vi "tcsWEP_logEvent_loopTimeOutOfRange.vi"(8 "error in (no error)":errorcluster, 11 "logevent_loopTimeOutOfRange_Ctl":T1) -> (0 "error out":errorcluster, 2 "function return":i32, 3 "logevent_loopTimeOutOfRange_Ctl out":T1)   [LabVIEW 2016, in "SALLV_tcsWEP.lvlib"]
doc: "int tcsWEP_shm_logEvent_loopTimeOutOfRangeLV(tcsWEP_logevent_loopTimeOutOfRangeLV *logevent_loopTimeOutOfRange_Ctl );"
uses:
  SALLV_tcsWEP.lvlib
  DataTypes/logevent_loopTimeOutOfRange.ctl
  SALLV_tcsWEP.so
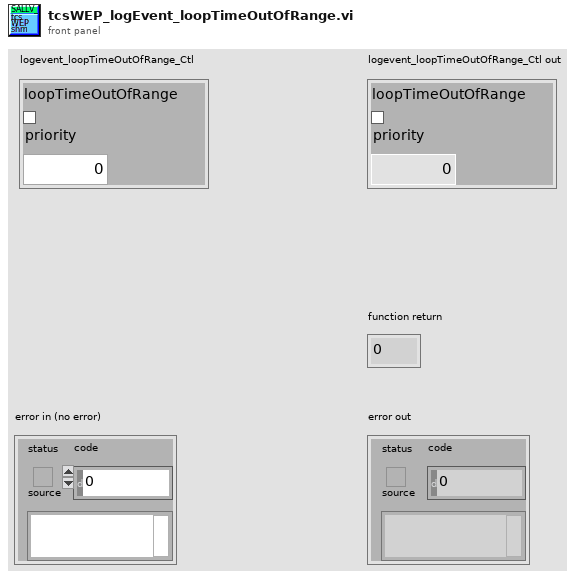
[diagram p1: front panel]
types:
  T1 = typedef "SALLV_tcsWEP.lvlib/logevent_loopTimeOutOfRange.ctl" = cluster{"loopTimeOutOfRange":bool, "priority":i32}
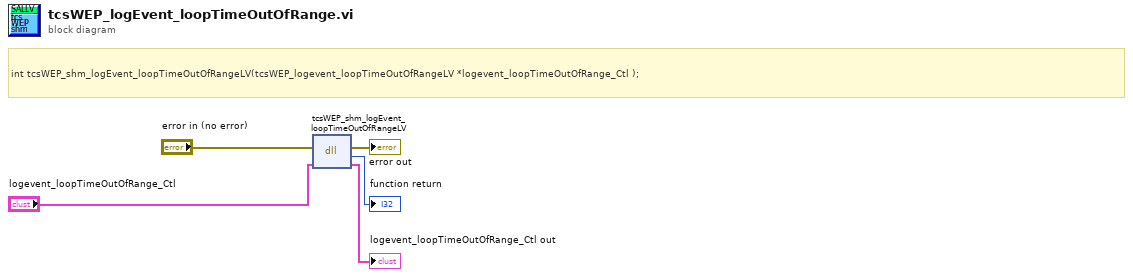
[diagram p0: block diagram]
diagram:
  # "int tcsWEP_shm_logEvent_loopTimeOutOfRangeLV(tcsWEP_logevent_loopTimeOutOfRangeLV *logevent_loopTimeOutOfRange_Ctl );"
  n1 = dll-call lib="home/ttsai/Documents/salAPI/SALLV_tcsWEP.*" fn="tcsWEP_shm_logEvent_loopTimeOutOfRangeLV"(error in="error in (no error)", "logevent_loopTimeOutOfRange_Ctl"="logevent_loopTimeOutOfRange_Ctl") -> (error out=→"error out":errorcluster, →"function return":i32, "logevent_loopTimeOutOfRange_Ctl"=→"logevent_loopTimeOutOfRange_Ctl out":T1)  [unwired: 2 in, 1 out]
